vi "PopUp.vi"(8 "error in (no error)":errorcluster, 10 "Message":string, 11 "Hello World in":refnum<class "Hello World.lvclass">) -> (0 "error out":errorcluster, 3 "Hello World out":refnum<class "Hello World.lvclass">)   [LabVIEW 2021, in "Hello World.lvlib" / "Hello World.lvclass"]
uses:
  Hello World.lvclass
  Hello World.lvclass/Hello World.ctl
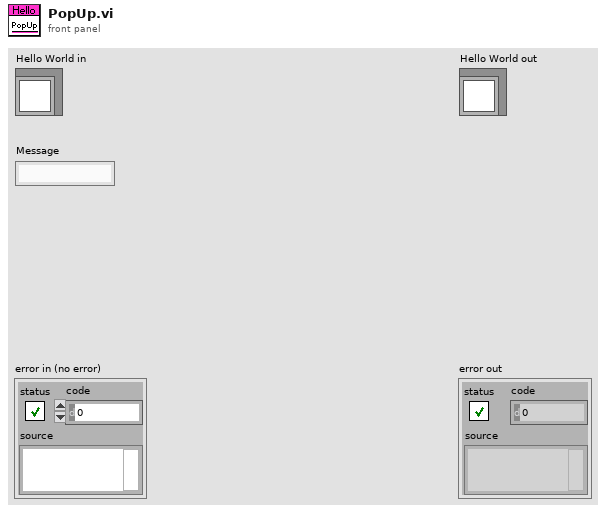
[diagram p1: front panel]
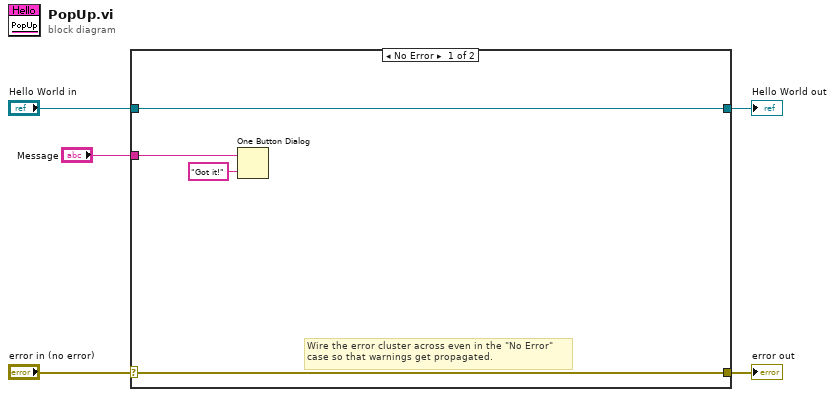
[diagram p0: block diagram]
diagram:
  n1 = case shown="No Error" "error in (no error)" {
    selector: "error in (no error)" -> [w8 w11]
    tunnel: [w8 w11] -> w4
    tunnel: [w9 w10] -> w2
    tunnel: "Hello World in" -> [w9 w10]
    tunnel: "Message" -> [w7 _]
    frame No Error {
      # "Wire the error cluster across even in the \"No Error\"\ncase so that warnings get propagated."
      n2 = One Button Dialog(message=w7, button name ("OK")="Got it!") -> ()  [unwired: 1 out]
    }
    frame Error {
    }
  }
  "error out" <- w4
  "Hello World out" <- w2
